vi "attachments.get.vi"(8 "error in (no error)":errorcluster, 11 "asset in":refnum<class "asset.lvclass">) -> (0 "error out":errorcluster, 2 "attachments":string[](array[string]), 3 "asset out":refnum<class "asset.lvclass">)   [LabVIEW 2020, in "asset.lvclass"]
uses:
  asset.lvclass
  asset.lvclass/asset.ctl
  nominal types/labels/labels.lvclass
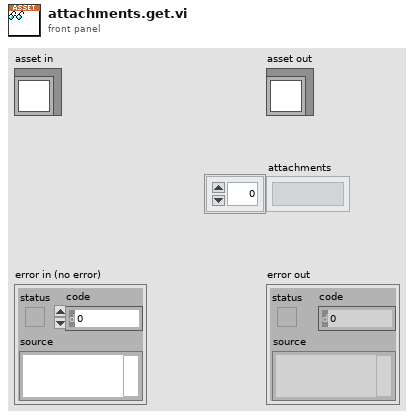
[diagram p1: front panel]
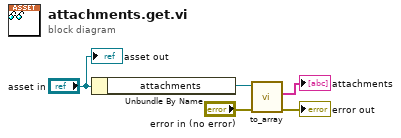
[diagram p0: block diagram]
diagram:
  n1 = Unbundle By Name("asset in") -> ("attachments"=w1:refnum<class "labels.lvclass">)
  n2 = call "to_array.vi"("error in"="error in (no error)", "labels in"=w1) -> ("error out"=→"error out":errorcluster, "Labels Array"=→"attachments":string[])  [unwired: 7 in, 1 out]
  "asset out" <- "asset in"
